vi "Base Directory.vi"(6 "Operation":T1, 8 "Error In":errorcluster) -> (0 "Error Out":errorcluster, 3 "Base Directory":path)   [LabVIEW 2016]
uses:
  Save Trace/Global Variable Control.ctl
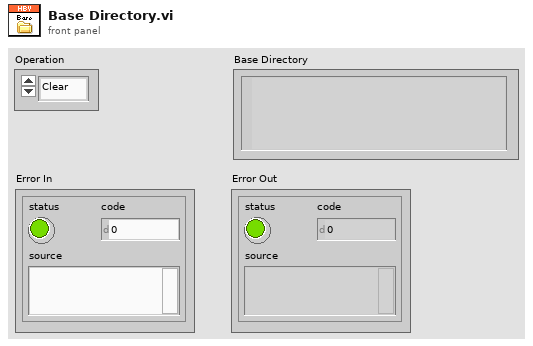
[diagram p1: front panel]
types:
  T1 = typedef "Global Variable Control.ctl" = enum16{"Clear", "Set", "Get"}
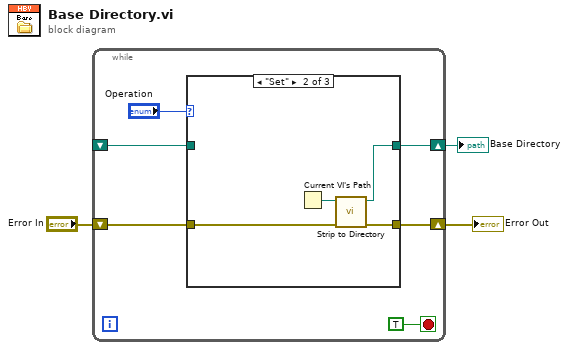
[diagram p0: block diagram]
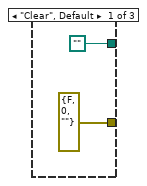
[diagram p2: hidden frame]
diagram:
  n1 = while {
    shift-right: [w7] -> w3
    shift-left: _ -> [w6]
    shift-right: [w5] -> w2
    shift-left: "Error In" -> [w4]
    stop <- TRUE stop-if-true
    n2 = case shown="\"Set\"" "Operation" {
      tunnel: [path "" w13 w17] -> w7
      tunnel: w6 -> [_ _ w17]
      tunnel: [errorcluster {"status"=FALSE, "code"=0, "source"=""} ("Error Out 2") w14 w16] -> w5
      tunnel: w4 -> [_ w15 w16]
      frame "Clear", Default {
      }
      frame "Set" {
        n3 = Current VI's Path() -> (path=w12:path)
        n4 = call "Strip to Directory.vi"("Error In"=w15, "Path in"=w12) -> ("Error Out"=w14:errorcluster, "Directory Out"=w13:path)  [unwired: 8 in]
      }
      frame "Get" {
      }
    }
  }
  "Base Directory" <- w3
  "Error Out" <- w2
